vi "Wait Until Com.vi"(1 "command text in":string[](array[string]), 2 "Data Acq":T4=enum."NML Data Acquisition-New.vi", 3 "option":T2) -> (0 "Command text out":string[][](array[string]))   [LabVIEW 2019]
uses:
  Ctl/Data Acquisition System.ctl
  Wait Until.ctl
  Wait Until condition.ctl
  Ctl/option.ctl
panel:
  in  "initial wait (sec)":dbl=10.0
  out "selected index 2":u32
  in  "Timeout (sec)":dbl=30000.0
  in  "xxx%":dbl
  in  "wait Condition":T1=enum."= target value"
  in  "Target Value":dbl
  in  "Available Data":string[](array[string])
  in  "cancel":bool
  in  "enter":bool
  in  "Wait Until Ctr":T3={"Available Data"=[], "Target Value"=0.0, "Condition"=enum."= target value", "xxx%"=0.0, "Timeout (sec)"=30000.0, "selected index"=0, "initial wait (sec)"=0.0}
  out "error out 2":errorcluster
  out "error out":errorcluster
  # "Wait Until Command"
  # "This command waits until 'DATA' value in NML Data Acquisition program meets user specified the condition."
  # "Select DATA to monitor"
  # "Enter Target value"
  # "Initial wait before 'condition' applies:"
  # "sec"
  # "Specifiy 'wait until' condition"
  # "Wait until DATA  is"
  # "(Specify"
  # "if necessary)"
  # "Enter 'Time out' here"
  # "sec"
  # "Wait Until Command"
  # "This command waits until 'DATA' value in NML Data Acquisition program meets user specified the condition."
  # "Select DATA to monitor"
  # "Enter Target value"
  # "Specifiy 'wait until' condition"
  # "Wait until DATA  is"
  # "(Specify"
  # "if necessary)"
  # "Enter 'Time out' here"
  # "sec"
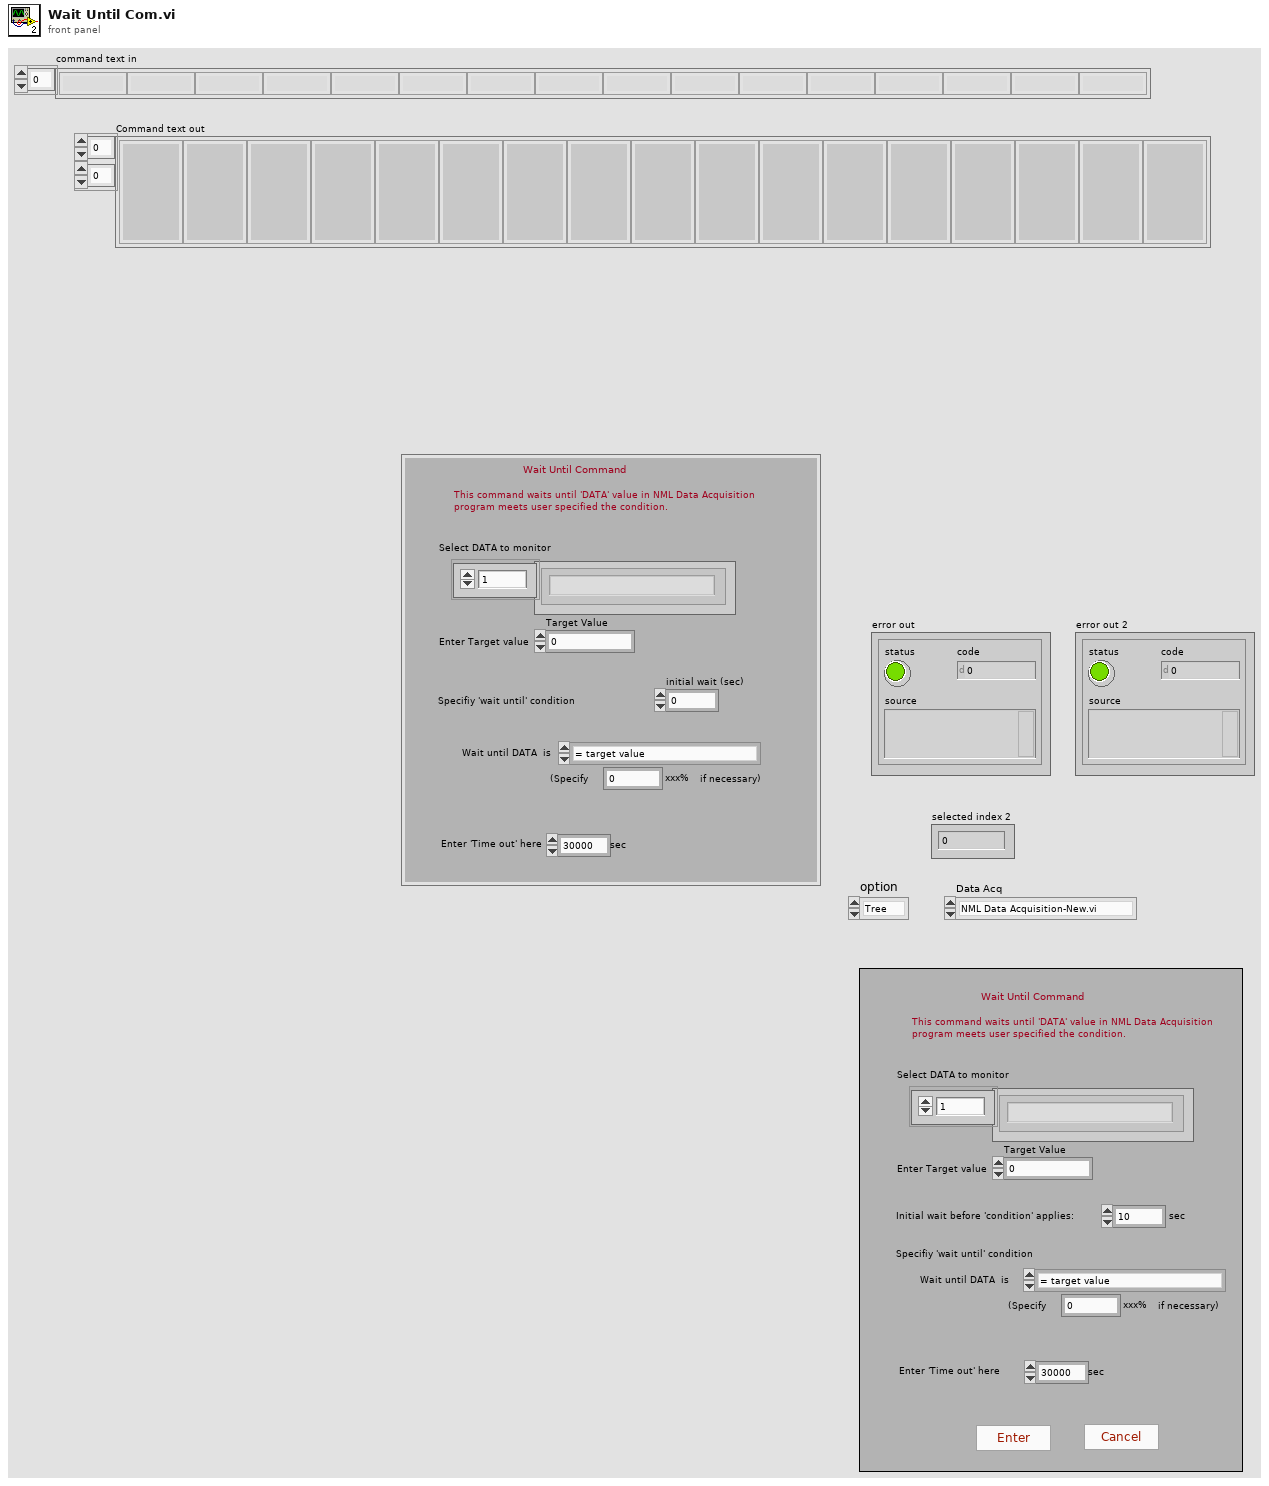
[diagram p1: front panel]
types:
  T1 = typedef "Wait Until condition.ctl" = enum16{"within xxx% of target value", "<= target value", ">= target value", "= target value"}
  T2 = typedef "option.ctl" = enum16{"Tree", "List"}
  T3 = typedef "Wait Until.ctl" = cluster{"Available Data":string[], "Target Value":dbl, "Condition":T1, "xxx%":dbl, "Timeout (sec)":dbl, "selected index":u32, "initial wait (sec)":dbl}
  T4 = typedef "Data Acquisition System.ctl" = enum16{"NML Data Acquisition-old.vi", "NML Data Acquisition-New.vi"}
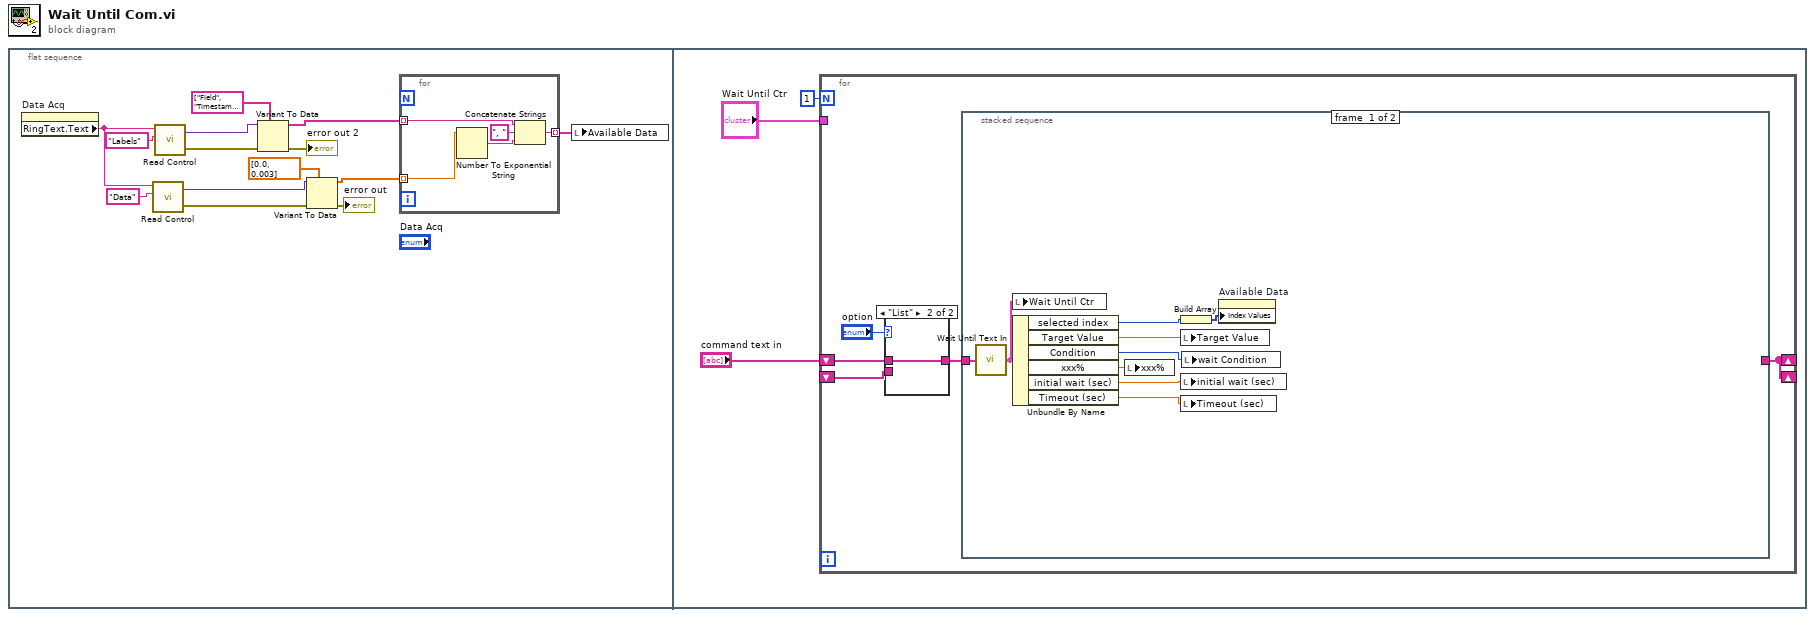
[diagram p0: block diagram]
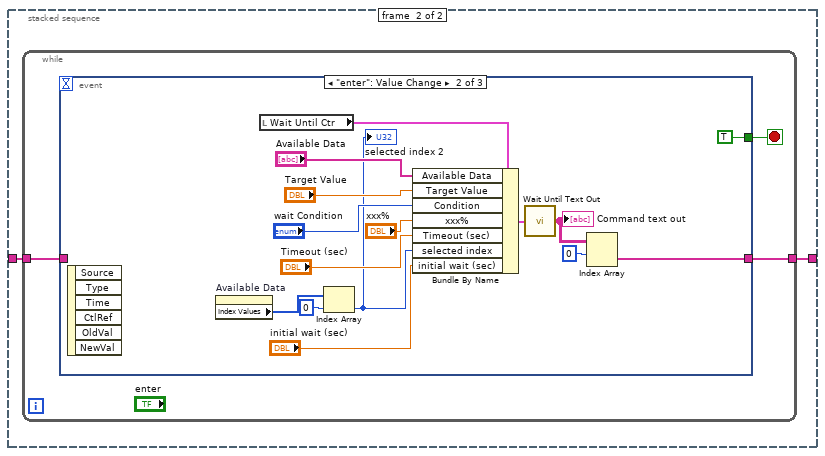
[diagram p2: hidden frame]
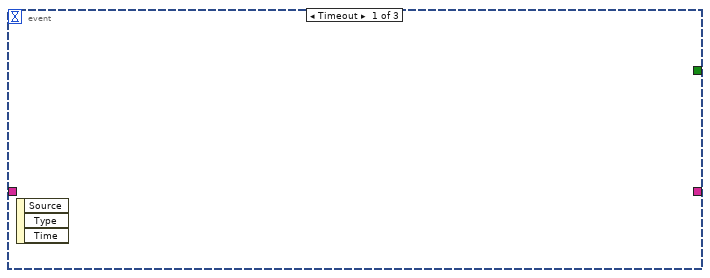
[diagram p3: hidden frame]
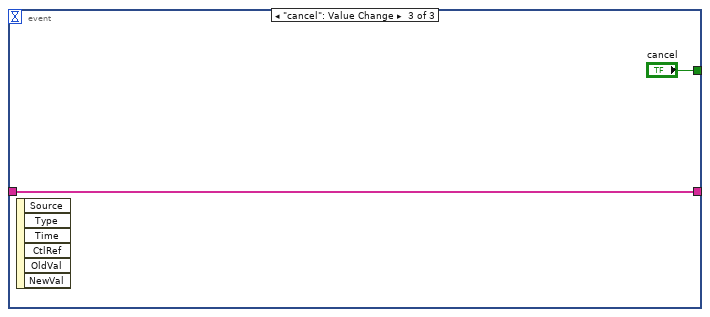
[diagram p4: hidden frame]
diagram:
  n1 = flat-sequence {
    frame #0 {
      n2 = property on="Data Acq" class="Enum (strict)"() -> ("RingText.Text"=w1:string)  [unwired: 2 in, 2 out]
      n3 = call "Read Control.vi"("VI Name"=w1, "Control Name"="Data") -> ("Value"=w8:variant, "error out"=w2:errorcluster)  [unwired: 3 in]
      n4 = call "Read Control.vi"("VI Name"=w1, "Control Name"="Labels") -> ("Value"=w9:variant, "error out"=w3:errorcluster)  [unwired: 3 in]
      n5 = Variant To Data(error in=w3, type=string[] ["Field", "Timestamp"] ("Labels"), Variant=w9) -> (data=w12:string[], error out=→"error out 2":errorcluster)
      n6 = Variant To Data(error in=w2, type=dbl[] [0.0, 0.003] ("Data"), Variant=w8) -> (data=w13:dbl[], error out=→"error out":errorcluster)
      n7 = for {
        tunnel: w12 -> [w18] mode=indexing
        tunnel: w13 -> [w19] mode=indexing
        tunnel: [w15] -> w14 mode=indexing
        n8 = Number To Exponential String(number=w19) -> (E-format string=w16:string)  [unwired: 3 in]
        n9 = Concatenate Strings(w18, ", " ("string"), w16) -> (w15:string)
      }
      n10 = local write "Available Data"(w14) -> ()
    }
    frame #1 {
      n11 = for {
        N: 1 -> [_]
        tunnel: "Wait Until Ctr" -> [_]
        shift-right: [w23] -> _
        shift-left: "command text in" -> [w26]
        shift-right: [w23] -> _
        shift-left: _ -> [w24]
        n12 = case shown="\"List\"" "option" {
          tunnel: [w59 w60] -> w25
          tunnel: w26 -> [_ w60]
          tunnel: w24 -> [w59 _]
          frame "Tree", Default {
          }
          frame "List" {
          }
        }
        n13 = stacked-sequence {
          tunnel: w25 -> [w36 w37]
          tunnel: [_ w38] -> w23
          frame #0 {
            n14 = call "Wait Until Text In.vi"("command text in"=w36) -> ("Wait Until Ctr"=w35:T3)
            n15 = local write "Wait Until Ctr"(w35) -> ()
            n16 = Unbundle By Name(w35) -> ("selected index"=w34:u32, "Target Value"=w31:dbl, "Condition"=w32:T1, "xxx%"=w28:dbl, "initial wait (sec)"=w29:dbl, "Timeout (sec)"=w30:dbl)
            n17 = local write "xxx%"(w28) -> ()
            n18 = Build Array(w34) -> (w33:u32[])
            n19 = local write "Target Value"(w31) -> ()
            n20 = local write "initial wait (sec)"(w29) -> ()
            n21 = local write "Timeout (sec)"(w30) -> ()
            n22 = local write "wait Condition"(w32) -> ()
            n23 = property on="Available Data" class="Arr (strict)"("Index Values"=w33) -> ()  [unwired: 2 in, 2 out]
          }
          frame #1 {
            n24 = while {
              tunnel: [w41] -> w38
              tunnel: w37 -> [w39]
              stop <- w40 stop-if-true
              n25 = event shown="[1] \"enter\": Value Change" {
                selector: _ -> [_ _ _]
                dyn-events: _ -> [_ _ _]
                timeout: _ -> [_ _ _]
                tunnel: [_ w54 w58] -> w41
                tunnel: [_ TRUE "cancel"] -> w40
                tunnel: w39 -> [_ _ w58]
                event Timeout {
                  n26 = event-data() -> ()  [unwired: 1 in, 3 out]
                }
                event "enter": Value Change {
                  n27 = event-data() -> ()  [unwired: 1 in, 6 out]
                  n28 = property on="Available Data" class="Arr (strict)"() -> ("Index Values"=w45:u32[])  [unwired: 2 in, 2 out]
                  n29 = local read "Wait Until Ctr"() -> (w52:T3)
                  n30 = Index Array(array=w45, index=0) -> (element=w43:u32)
                  "selected index 2" <- w43
                  n31 = Bundle By Name(cluster=w52, "Available Data"="Available Data", "Target Value"="Target Value", "Condition"="wait Condition", "xxx%"="xxx%", "Timeout (sec)"="Timeout (sec)", "selected index"=w43, "initial wait (sec)"="initial wait (sec)") -> (w51:T3)
                  n32 = call "Wait Until Text Out.vi"("Wait Until Ctr"=w51) -> ("Command text"=w55:string[][])
                  "Command text out" <- w55
                  n33 = Index Array(array=w55, index (row)=0 ("disabled index (col)")) -> (element=w54:string[])  [unwired: 1 in]
                }
                event "cancel": Value Change {
                  n34 = event-data() -> ()  [unwired: 1 in, 6 out]
                }
              }
            }
          }
        }
      }
    }
  }
